vi "Configure Read LabVIEW Measurement File.vi"(0 "subVI":refnum<vi>, 2 "VI":refnum<vi>, 3 "ParentVI":refnum<vi>) -> (1 "Data Valid":bool)   [LabVIEW 2017]
doc: "Reads data from a text-based measurement file (.lvm) or binary measurement file (.tdm or .tdms)."
uses:
  <vilib>/express/express shared/ExFile.llb/ex_FileFormats.ctl
  <vilib>/express/express input/ExFileReadBlock.llb/ex_RetrieveParams.ctl
  <vilib>/express/express input/ExFileReadBlock.llb/ex_ReadFileGenericParams.ctl
  <vilib>/express/express shared/ExFile.llb/ex_FileGlobals.vi
panel:
  in  "Samples":i32=1 min=1
  in  "Segment Size":T1
  in  "Read generic text files":bool
  in  "Streaming":bool
  in  "Retrieve single values":bool
  in  "always hostless warning":string="The current target will not have a host computer connected.  When you run this VI, it will return an error."
  in  "maybe hostless warning":string="The current target might not always have a host connected.  When you run this VI with no host connected, it will return an error."
  in  "delimiter string":string
  in  "absolute time":bool
  in  "relative time?":bool
  in  "Decimal point":enum32{". (dot)", ", (comma)"}(radio)
  in  "Delimiter":enum32{"tab", "comma"}(radio)
  in  "storage_format":T2
  in  "Filename":path=path "test.lvm"
  in  "File path":path
  in  "Unable to Load":string="Unable to Read from File"
  in  "Generic Params":T3
  in  "Read File Now":bool
  out "Sample data":string[][](table)
  in  "First column is time channel":bool
  in  "First row is channel names":bool
  in  "Start row of numeric data":i32=1 min=1
  in  "Help":bool
  in  "Ok":bool
  in  "Cancel":bool
  in  "Retrieve segments of specified size":bool
  in  "Ask user to choose file":bool
  # "Filename"
  # "Time Stamps"
  # "File Format"
  # "Action"
  # "Generic Text File"
  # "Delimiter"
  # "Decimal Point"
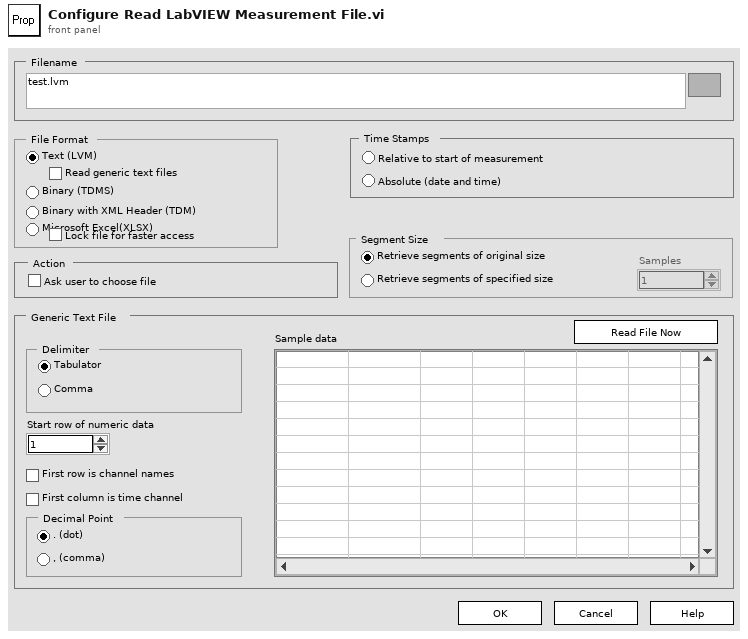
[diagram p1: front panel]
types:
  T1 = typedef "ex_RetrieveParams.ctl" = enum32{"Retrieve segments of original size", "Retrieve segments of specified size"}
  T2 = typedef "ex_FileFormats.ctl" = enum32{"lvm", "tdm", "tdms", "xlsx"}
  T3 = typedef "ex_ReadFileGenericParams.ctl" = cluster{"Delimiter":string, "First Row is Channel Names":bool, "First Column is Time Channel":bool, "Decimal Point":i32, "Start Row":i32}
  T4 = cluster{"Ctl Type":u16, "LV Block Ctl Label":string, "Wizard Ctl Label":string}[]
  T5 = typedef "propPageData.ctl" = cluster{"InstanceCtlRefs":refnum<vi>[], "ConfigDlgCtlRefs":refnum<vi>[], "Control Data":cluster{"Ctl Type":u16, "Instance Ctl Label":string, "Config Dialog Ctl Label":string}[], "viref Instance":refnum<vi>, "Types":i32[], "Config DialogVI":refnum<vi>}
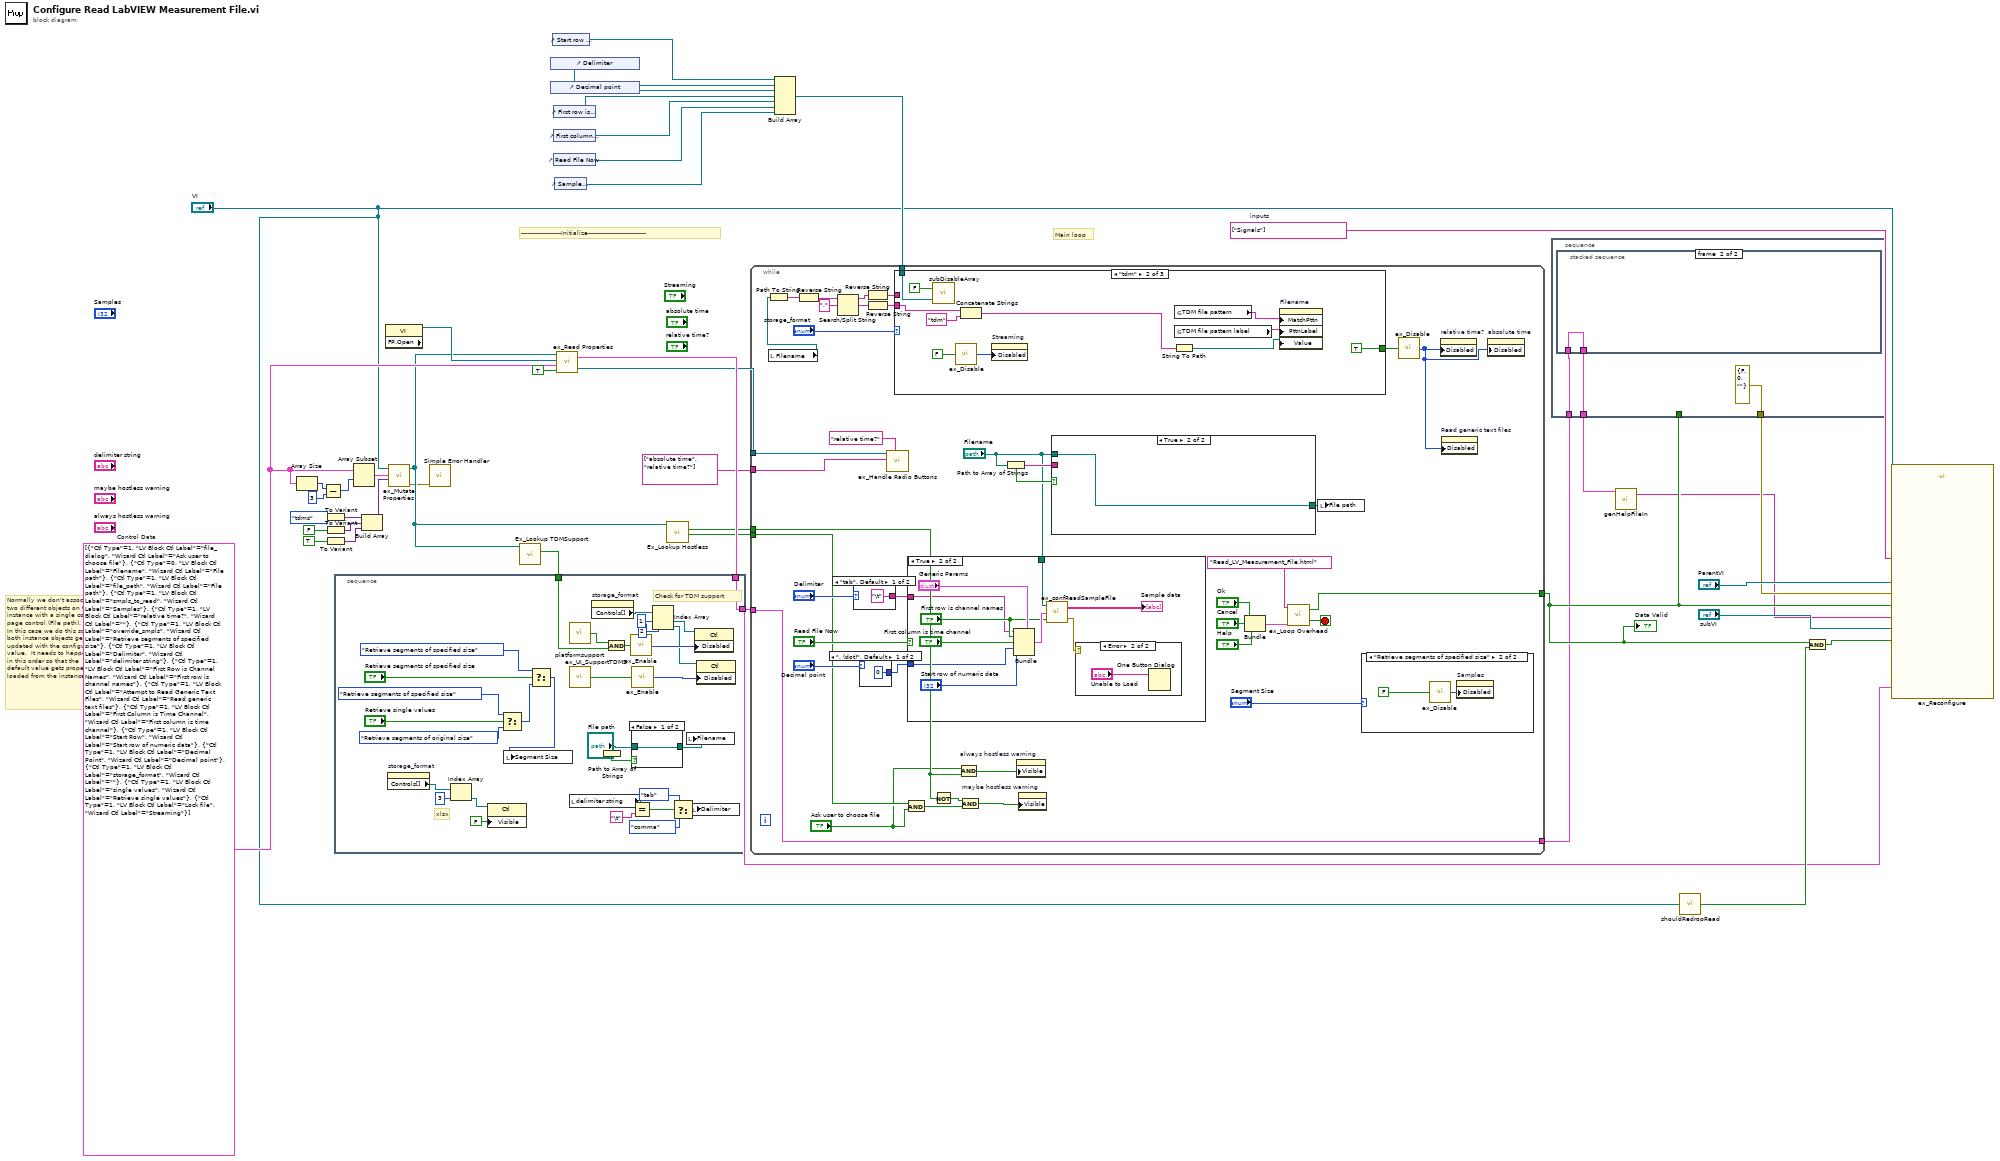
[diagram p0: block diagram]
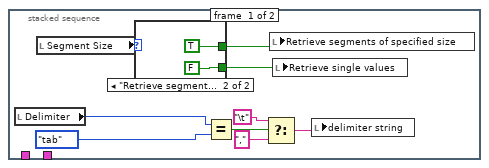
[diagram p2: hidden frame]
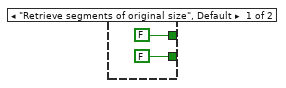
[diagram p3: hidden frame]
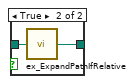
[diagram p4: hidden frame]
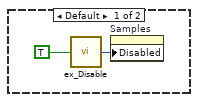
[diagram p5: hidden frame]
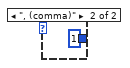
[diagram p6: hidden frame]
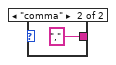
[diagram p7: hidden frame]
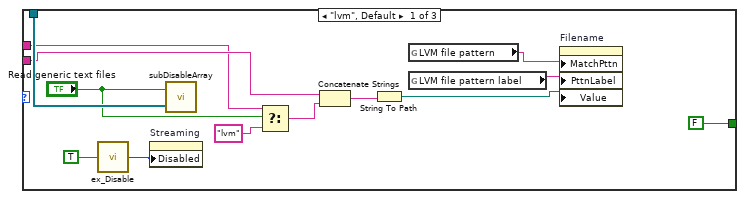
[diagram p8: hidden frame]
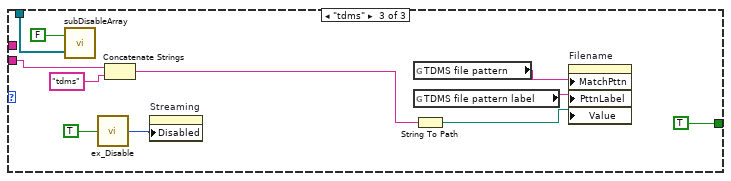
[diagram p9: hidden frame]
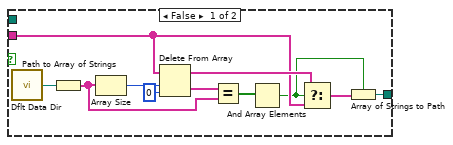
[diagram p10: hidden frame]
diagram:
  w28 = string[] ["Signals"]  # inputs
  w24 = T4 [{"Ctl Type"=1, "LV Block Ctl Label"="file_dialog", "Wizard Ctl Label"="Ask user to choose file"}, {"Ctl Type"=0, "LV Block Ctl Label"="Filename", "Wizard Ctl Label"="File path"}, {"Ctl Type"=1, "LV Block Ctl Label"="file_path", "Wizard Ctl Label"="File path"}, {"Ctl Type"=1, "LV Block Ctl Label"="smpls_to_read", "Wizard Ctl Label"="Samples"}, {"Ctl Type"=1, "LV Block Ctl Label"="relative time?", "Wizard Ctl Label"=""}, {"Ctl Type"=1, "LV Block Ctl Label"="override_smpls", "Wizard Ctl Label"="Retrieve segments of specified size"}, {"Ctl Type"=1, "LV Block Ctl Label"="Delimiter", "Wizard Ctl Label"="delimiter string"}, {"Ctl Type"=1, "LV Block Ctl Label"="First Row is Channel Names", "Wizard Ctl Label"="First row is channel names"}, {"Ctl Type"=1, "LV Block Ctl Label"="Attempt to Read Generic Text Files", "Wizard Ctl Label"="Read generic text files"}, {"Ctl Type"=1, "LV Block Ctl Label"="First Column is Time Channel", "Wizard Ctl Label"="First column is time channel"}, {"Ctl Type"=1, "LV Block Ctl Label"="Start Row", "Wizard Ctl Label"="Start row of numeric data"}, {"Ctl Type"=1, "LV Block Ctl Label"="Decimal Point", "Wizard Ctl Label"="Decimal point"}, {"Ctl Type"=1, "LV Block Ctl Label"="storage_format", "Wizard Ctl Label"=""}, {"Ctl Type"=1, "LV Block Ctl Label"="single values", "Wizard Ctl Label"="Retrieve single values"}, {"Ctl Type"=1, "LV Block Ctl Label"="Lock file", "Wizard Ctl Label"="Streaming"}]  # Control Data
  # "Normally we don't associate\ntwo different objects on the\ninstance with a single config\npage control (File path).\nIn this case we do this so\nboth instance objects get\nupdated with the configured\nvalue.  It needs to happen\nin this order so that the\ndefault value gets properly\nloaded from the instance."
  # "--------------------Initialize-----------------------------"
  # "Main loop"
  n1 = Array Size(array=w24) -> (size(s)=w20:i32)
  n2 = Subtract(x=w20, y=3) -> (x-y=w18:i32)
  n3 = To Variant(anything=ex_FileFormats."tdms" ("storage_format")) -> (Variant=w15:variant)
  n4 = To Variant(anything=FALSE) -> (Variant=w13:variant)
  n5 = To Variant(anything=TRUE) -> (Variant=w11:variant)
  n6 = Array Subset(array=w24, index=w18) -> (w17:T4)  [unwired: 1 in]
  n7 = Build Array(w15, w13, w11) -> (w14:variant[])
  n8 = property class="VI" props=["FP.Open"]() -> (reference out=w42:refnum<vi>)  [unwired: 2 in, 2 out]
  n9 = call <vilib>:"ex_Mutate Properties.vi"("Control Values"=w14, "Control Data"=w17, "VI ref in"="VI") -> ("error out"=w9:errorcluster, "VI ref out"=w23:refnum<vi>)  [unwired: 7 out]
  n10 = call <vilib>:"Simple Error Handler.vi"("error in (no error)"=w9) -> ()  [unwired: 1 in, 8 out]
  n11 = call <vilib>:"Ex_Lookup TDMSupport.vi"("VI RefNum for Context"=w23) -> ("TDM Support?"=w22:bool)  [unwired: 1 in, 9 out]
  n12 = control-ref of="Delimiter"() -> (w33:refnum<vi>)
  n13 = control-ref of="Decimal point"() -> (w34:refnum<vi>)
  n14 = control-ref of="Start row of numeric data"() -> (w32:refnum<vi>)
  n15 = control-ref of="First row is channel names"() -> (w38:refnum<vi>)
  n16 = control-ref of="First column is time channel"() -> (w37:refnum<vi>)
  n17 = control-ref of="Read File Now"() -> (w36:refnum<vi>)
  n18 = control-ref of="Sample data"() -> (w35:refnum<vi>)
  n19 = call <vilib>:"ex_Read Properties.vi"("Ignore Errors"=TRUE, "Control Data"=w24, "viref Configuration Dialog"=w42, "viref Instance"=w23) -> ("viref Configuration Dialog out"=w31:refnum<vi>, "Output Cluster"=w39:T5)  [unwired: 2 out]
  n20 = stacked-sequence {
    tunnel: w39 -> [w74]
    tunnel: [w74] -> w4
    tunnel: w22 -> [w52]
    frame #0 {
      # "xlsx"
      # "Check for TDM support"
      n21 = property on="storage_format" class="RadioBtnsControl (strict)"() -> ("Controls[]"=w43:refnum<vi>[])  [unwired: 2 in, 2 out]
      n22 = Index Array(array=w43, index=3) -> (element=w45:refnum<vi>)
      n23 = property class="Ctl"(reference=w45, "Visible"=FALSE) -> ()  [unwired: 1 in, 2 out]
      n24 = Select(t=ex_RetrieveParams."Retrieve segments of specified size" ("Segment Size"), s="Retrieve single values", f=ex_RetrieveParams."Retrieve segments of original size" ("Segment Size")) -> (s? t:f=w58:T1)
      n25 = Select(t=ex_RetrieveParams."Retrieve segments of specified size" ("Segment Size"), s="Retrieve segments of specified size", f=w58) -> (s? t:f=w54:T1)
      n26 = local write "Segment Size"(w54) -> ()
      n27 = call <vilib>:"platformsupport.vi"() -> ("TDM Support for Platform"=w53:bool)  [unwired: 1 out]
      n28 = call <vilib>:"ex_UI_SupportTDMS.vi"() -> ("support TDMSû"=w47:bool)  [unwired: 2 in]
      n29 = local read "delimiter string"() -> (w61:string)
      n30 = property on="storage_format" class="RadioBtnsControl (strict)"() -> ("Controls[]"=w70:refnum<vi>[])  [unwired: 2 in, 2 out]
      n31 = Path to Array of Strings(0:"File path") -> (1:w72:bool)  [unwired: 1 out]
      n32 = And(x=w53, y=w52) -> (x .and. y?=w49:bool)
      n33 = call <vilib>:"ex_Enable.vi"("Enable?"=w49) -> ("Disabled Value"=w69:u8)
      n34 = Equal?(x=w61, y="\t") -> (x = y?=w65:bool)
      n35 = call <vilib>:"ex_Enable.vi"("Enable?"=w47) -> ("Disabled Value"=w48:u8)
      n36 = case shown="False" w72 {
        tunnel: "File path" -> [w75 w77]
        tunnel: [w75 w76] -> w73
        frame False {
        }
        frame True {
          n37 = call <vilib>:"ex_ExpandPathIfRelative.vi"("Path"=w77) -> ("Expanded path"=w76:path)  [unwired: 4 out]
        }
      }
      n38 = Index Array(array=w70, index #1=1 ("index"), index #2=2 ("index")) -> (element #1=w68:refnum<vi>, element #2=w50:refnum<vi>)
      n39 = Select(t=enum32{"tab", "comma"}."tab" ("Delimiter"), s=w65, f=enum32{"tab", "comma"}."comma" ("Delimiter")) -> (s? t:f=w64:enum32{"tab", "comma"})
      n40 = local write "Filename"(w73) -> ()
      n41 = local write "Delimiter"(w64) -> ()
      n42 = property class="Ctl"(reference=w68, "Disabled"=w69) -> ()  [unwired: 1 in, 2 out]
      n43 = property class="Ctl"(reference=w50, "Disabled"=w48) -> ()  [unwired: 1 in, 2 out]
    }
  }
  n44 = call <vilib>:"Ex_Lookup Hostless.vi"("VI RefNum for Context"=w23) -> ("Maybe Hostless"=w25:bool, "Always Hostless"=w26:bool)  [unwired: 1 in, 8 out]
  n45 = Build Array(w32, w33, w34, w38, w37, w36, w35) -> (w29:refnum<vi>[])
  n46 = while {
    tunnel: [w116] -> w5
    tunnel: w31 -> [w98]
    tunnel: string[] ["absolute time", "relative time?"] -> [w99]
    tunnel: w4 -> [w78]
    tunnel: w29 -> [w97]
    tunnel: w25 -> [w90]
    tunnel: w26 -> [w89]
    tunnel: [w78] -> w2
    stop <- w115 stop-if-true
    n47 = local read "Filename"() -> (w82:path)
    n48 = Path To String(path=w82) -> (string=w86:string)
    n49 = Reverse String(1:w86) -> (0:w85:string)
    n50 = Search/Split String(string=w85, search string/char (-)=".") -> (substring before match=w80:string, match + rest of string=w83:string)  [unwired: 2 out]
    n51 = case shown="\"tab\", Default" "Delimiter" {
      tunnel: ["\t" ","] -> w103
      frame "tab", Default {
      }
      frame "comma" {
      }
    }
    n52 = case shown="\". (dot)\", Default" "Decimal point" {
      tunnel: [0 1] -> w101
      frame ". (dot)", Default {
      }
      frame ", (comma)" {
      }
    }
    n53 = Reverse String(1:w80) -> (0:w79:string)
    n54 = Reverse String(1:w83) -> (0:w81:string)
    n55 = call <vilib>:"ex_Handle Radio Buttons.vi"("Boolean Control"="relative time?", "Radio Buttons"=w99, "VI refnum"=w98) -> ()  [unwired: 4 in, 5 out]
    n56 = case shown="\"tdm\"" "storage_format" {
      tunnel: w97 -> [w135 w146 w157]
      tunnel: [FALSE ("Disable?") TRUE ("Disable?") TRUE ("Disable?")] -> w96
      tunnel: w81 -> [w130 w141 w152]
      tunnel: w79 -> [w127 _ _]
      frame "lvm", Default {
        n57 = call <vilib>:"ex_Disable.vi"("Disable?"=TRUE) -> ("Disabled value"=w133:u8)
        n58 = property on="Streaming" class="Bool (strict)"("Disabled"=w133) -> ()  [unwired: 2 in, 2 out]
        n59 = call <vilib>:"subDisableArray.vi"("Array"=w135, "Enable"="Read generic text files") -> ()
        n60 = Select(t=w127, s="Read generic text files", f="lvm" ("replace string (\"\")")) -> (s? t:f=w128:string)
        n61 = Concatenate Strings(w130, w128) -> (w131:string)
        n62 = String To Path(string=w131) -> (path=w136:path)
        n63 = global read "ex_FileGlobals.vi" "LVM file pattern"() -> (w138:string)
        n64 = global read "ex_FileGlobals.vi" "LVM file pattern label"() -> (w137:string)
        n65 = property on="Filename" class="Path"("MatchPttn"=w138, "PttnLabel"=w137, "Value"=w136) -> ()  [unwired: 2 in, 2 out]
      }
      frame "tdm" {
        n66 = call <vilib>:"subDisableArray.vi"("Array"=w146, "Enable"=FALSE) -> ()
        n67 = call <vilib>:"ex_Disable.vi"("Disable?"=FALSE) -> ("Disabled value"=w143:u8)
        n68 = Concatenate Strings(w141, "tdm" ("replace string (\"\")")) -> (w139:string)
        n69 = property on="Streaming" class="Bool (strict)"("Disabled"=w143) -> ()  [unwired: 2 in, 2 out]
        n70 = String To Path(string=w139) -> (path=w147:path)
        n71 = global read "ex_FileGlobals.vi" "TDM file pattern"() -> (w149:string)
        n72 = global read "ex_FileGlobals.vi" "TDM file pattern label"() -> (w148:string)
        n73 = property on="Filename" class="Path"("MatchPttn"=w149, "PttnLabel"=w148, "Value"=w147) -> ()  [unwired: 2 in, 2 out]
      }
      frame "tdms" {
        n74 = call <vilib>:"subDisableArray.vi"("Array"=w157, "Enable"=FALSE) -> ()
        n75 = call <vilib>:"ex_Disable.vi"("Disable?"=TRUE) -> ("Disabled value"=w154:u8)
        n76 = Concatenate Strings(w152, "tdms" ("replace string (\"\")")) -> (w150:string)
        n77 = property on="Streaming" class="Bool (strict)"("Disabled"=w154) -> ()  [unwired: 2 in, 2 out]
        n78 = global read "ex_FileGlobals.vi" "TDMS file pattern"() -> (w160:string)
        n79 = global read "ex_FileGlobals.vi" "TDMS file pattern label"() -> (w159:string)
        n80 = String To Path(string=w150) -> (path=w158:path)
        n81 = property on="Filename" class="Path"("MatchPttn"=w160, "PttnLabel"=w159, "Value"=w158) -> ()  [unwired: 2 in, 2 out]
      }
    }
    n82 = And(x=w90, y="Ask user to choose file") -> (x .and. y?=w92:bool)
    n83 = case shown="True" "Read File Now" {
      tunnel: "Filename" -> [_ w182]
      tunnel: w103 -> [_ w174]
      tunnel: w101 -> [_ w173]
      frame False {
      }
      frame True {
        n84 = Bundle(cluster="Generic Params", "Delimiter"=w174, "First Row is Channel Names"="First row is channel names", "First Column is Time Channel"="First column is time channel", "Decimal Point"=w173, "Start Row"="Start row of numeric data") -> (w180:T3)
        n85 = call <vilib>:"ex_confReadSampleFile.vi"("First Row is Channel Names"="First row is channel names", "Generic Params"=w180, "Expanded path"=w182) -> ("error out"=w175:errorcluster, "Sample Data"=→"Sample data":string[][])
        n86 = case shown="Error" w175 {
          frame No Error {
          }
          frame Error {
            n87 = One Button Dialog(message="Unable to Load") -> ()  [unwired: 2 out]
          }
        }
      }
    }
    n88 = Not(x=w89) -> (.not. x?=w91:bool)
    n89 = And(x="Ask user to choose file", y=w89) -> (x .and. y?=w93:bool)
    n90 = And(x=w91, y=w92) -> (x .and. y?=w94:bool)
    n91 = Path to Array of Strings(0:"Filename") -> (1:w107:bool, 2:w108:string[])
    n92 = property on="always hostless warning" class="Str"("Visible"=w93) -> ()  [unwired: 2 in, 2 out]
    n93 = property on="maybe hostless warning" class="Str"("Visible"=w94) -> ()  [unwired: 2 in, 2 out]
    n94 = case shown="True" w107 {
      tunnel: [w163 w172] -> w109
      tunnel: "Filename" -> [_ w172]
      tunnel: w108 -> [w162 _]
      frame False {
        n95 = call <vilib>:"Dflt Data Dir.vi"() -> ("App:Default Data Directory"=w164:path)
        n96 = Path to Array of Strings(0:w164) -> (2:w171:string[])  [unwired: 1 out]
        n97 = Array Size(array=w171) -> (size(s)=w165:i32)
        n98 = Delete From Array(array=w162, length=w165, index=0) -> (deleted portion=w170:string[], array with subset deleted=w169:string[])
        n99 = Equal?(x=w170, y=w171) -> (x = y?=w167:bool[])
        n100 = And Array Elements(Boolean array=w167) -> (logical AND=w161:bool)
        n101 = Select(t=w169, s=w161, f=w162) -> (s? t:f=w168:string[])
        n102 = Array of Strings to Path(0:w168, 1:w161) -> (2:w163:path)
      }
      frame True {
      }
    }
    n103 = Bundle("Ok"="Ok", "Cancel"="Cancel", "Help"="Help") -> (w111:cluster{"Ok":bool, "Cancel":bool, "Help":bool})  [unwired: 1 out]
    n104 = call <vilib>:"ex_Loop Overhead.vi"("Bottom Button Bar"=w111, "Help string to search for"="Read_LV_Measurement_File.html") -> ("Loop Terminator"=w115:bool, "Data Valid"=w116:bool)  [unwired: 1 in, 1 out]
    n105 = local write "File path"(w109) -> ()
    n106 = case shown="\"Retrieve segments of specified size\"" "Segment Size" {
      frame Default {
        n107 = call <vilib>:"ex_Disable.vi"("Disable?"=TRUE) -> ("Disabled value"=w119:u8)
        n108 = property on="Samples" class="DigNum (strict)"("Disabled"=w119) -> ()  [unwired: 2 in, 2 out]
      }
      frame "Retrieve segments of specified size" {
        n109 = call <vilib>:"ex_Disable.vi"("Disable?"=FALSE) -> ("Disabled value"=w121:u8)
        n110 = property on="Samples" class="DigNum (strict)"("Disabled"=w121) -> ()  [unwired: 2 in, 2 out]
      }
    }
    n111 = call <vilib>:"ex_Disable.vi"("Disable?"=w96) -> ("Disabled value"=w95:u8)
    n112 = property on="relative time?" class="Bool (strict)"("Disabled"=w95) -> ()  [unwired: 2 in, 2 out]
    n113 = property on="Read generic text files" class="Bool (strict)"("Disabled"=w95) -> ()  [unwired: 2 in, 2 out]
    n114 = property on="absolute time" class="Bool (strict)"("Disabled"=w95) -> ()  [unwired: 2 in, 2 out]
  }
  "Data Valid" <- w5
  n115 = stacked-sequence {
    tunnel: w5 -> [_]
    tunnel: [errorcluster {"status"=FALSE, "code"=0, "source"=""} ("error out")] -> w27
    tunnel: w2 -> [w185]
    tunnel: [w184] -> w1
    frame #0 {
      n116 = stacked-sequence {
        tunnel: w185 -> [_ w200]
        tunnel: [_ w200] -> w184
        frame #0 {
          n117 = local read "Delimiter"() -> (w193:enum32{"tab", "comma"})
          n118 = local read "Segment Size"() -> (w189:T1)
          n119 = case shown="\"Retrieve segments of specified size\"" w189 {
            tunnel: [FALSE TRUE] -> w188
            tunnel: [FALSE FALSE] -> w187
            frame "Retrieve segments of original size", Default {
            }
            frame "Retrieve segments of specified size" {
            }
          }
          n120 = Equal?(x=w193, y=enum32{"tab", "comma"}."tab" ("Delimiter")) -> (x = y?=w195:bool)
          n121 = Select(t="\t", s=w195, f=",") -> (s? t:f=w191:string)
          n122 = local write "Retrieve segments of specified size"(w188) -> ()
          n123 = local write "Retrieve single values"(w187) -> ()
          n124 = local write "delimiter string"(w191) -> ()
        }
        frame #1 {
        }
      }
    }
  }
  n125 = call <vilib>:"genHelpFileIn.vi"("Output Cluster"=w1) -> ("Help Description"=w3:string)  [unwired: 5 in]
  n126 = call <vilib>:"shouldRedropRead.vi"("VI"="VI") -> ("redrop?"=w8:bool)
  n127 = And(x=w5, y=w8) -> (x .and. y?=w6:bool)
  n128 = call <vilib>:"ex_Reconfigure.vi"("VI refnum"="VI", "Parent VI refnum"="ParentVI", "Data Valid"=w5, "subVI refnum"="subVI", "error in"=w27, "ReDrop VI"=w6, "Inputs/Outputs to Grow"=w28, "Props Cluster"=w4, "Configuration Description"=w3) -> ()  [unwired: 4 in, 15 out]
